vi "_FPGA_MSProcess_DataReader.vi"(0 "Read":bool) -> (1 "Element":u64, 2 "new data":bool)   [LabVIEW 2018]
uses:
  <vilib>/rvi/interface/RandomDataEmulation/niFpgaRandomDataHandleErrors.vi
  <vilib>/rvi/DataTransferAndStorage/Container/XNode/niFpgaContainer.xnode
  <vilib>/rvi/interface/RandomDataEmulation/nirviRandomDataFpgaReadWriteTemplate.vi
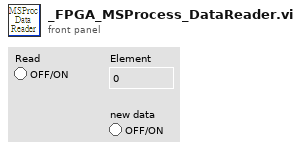
[diagram p1: front panel]
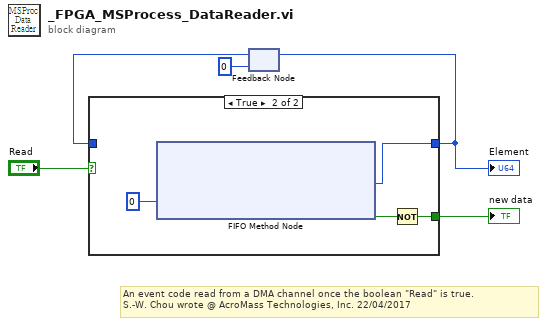
[diagram p0: block diagram]
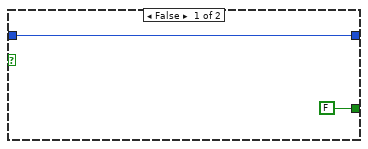
[diagram p2: hidden frame]
diagram:
  # "An event code read from a DMA channel once the boolean \"Read\" is true.\nS.-W. Chou wrote @ AcroMass Technologies, Inc. 22/04/2017"
  n1 = feedback #1(u64 0 ("Element")) -> (w2:u64)
  n2 = case shown="True" "Read" {
    tunnel: [FALSE w9] -> w4
    tunnel: [w6 w8] -> w3
    tunnel: w2 -> [w6 _]
    frame False {
    }
    frame True {
      n3 = xnode ("FIFO Method Node")("Timeout"=0) -> ("Element"=w8:u64, "Timed Out?"=w10:bool)  [unwired: 1 in, 1 out]
      n4 = Not(x=w10) -> (.not. x?=w9:bool)
    }
  }
  "new data" <- w4
  "Element" <- w3
  n5 = feedback-in #1(w3) -> ()
